vi "Read Rank.vi"(8 "error in (no error)":errorcluster, 11 "SA Path Group in":refnum<class "SA 18GHz Path Group.lvclass">) -> (0 "error out":errorcluster, 2 "Rank":dbl, 3 "SA Path Group out":refnum<class "SA 18GHz Path Group.lvclass">)   [LabVIEW 2023, in "RFFixtureCharact.RFPM.lvlib" / "SA 18GHz Path Group.lvclass"]
uses:
  SA 18GHz Path Group.lvclass
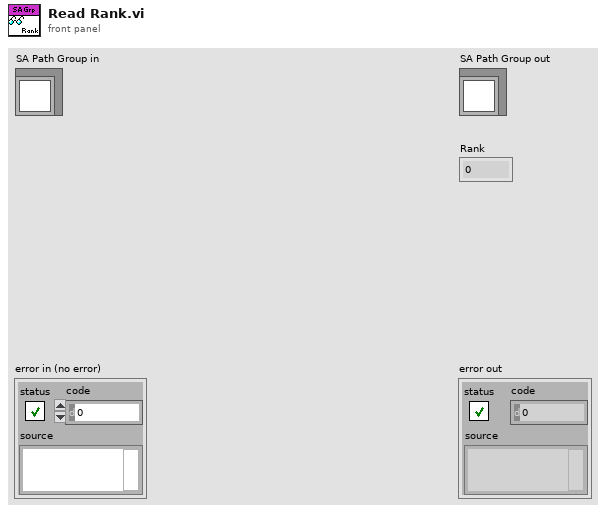
[diagram p1: front panel]
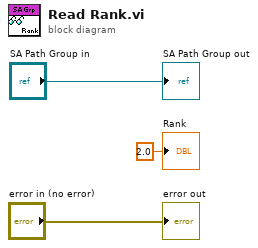
[diagram p0: block diagram]
diagram:
  "error out" <- "error in (no error)"
  "SA Path Group out" <- "SA Path Group in"
  "Rank" <- 2.0 ("Rank")
